vi "Agilent DSO1000 Series Acquire Multiple Waveforms.vi"() -> ()   [LabVIEW 2010]
doc: "This example shows how to configure multiple channels and acquire waveforms from multiple channels."
uses:
  <instrlib>/Agilent DSO1000 Series/Public/Data/Read Waveform (Multiple).vi
  <instrlib>/Agilent DSO1000 Series/Agilent DSO1000 Series.lvlib
panel:
  in  "Probe Attenuation (3: 1X)":u16(ring)=3 items=["0.001X", "0.01X", "0.1X", "1X", "10X", "100X", "1000X"]
  in  "Probe Attenuation (3: 1X)":u16(ring)=3 items=["0.001X", "0.01X", "0.1X", "1X", "10X", "100X", "1000X"]
  in  "Channel (1: Channel 1)":u16(ring)=2 items=["Channel 1"=1, "Channel 2"=2, "Channel 3"=3, "Channel 4"=4]
  in  "Channel (1: Channel 1)":u16(ring)=1 items=["Channel 1"=1, "Channel 2"=2, "Channel 3"=3, "Channel 4"=4]
  in  "Maximum Time (10000 ms)":u32=10000
  in  "Vertical Coupling (1: DC)":u16(ring)=1 items=["AC", "DC", "Ground"]
  in  "Vertical Coupling (1: DC)":u16(ring)=1 items=["AC", "DC", "Ground"]
  out "Waveform Data":waveform(dbl)[](graph)
  in  "VISA resource name":refnum<visa-resource-name>
  # "(c) 2009 National Instruments.  ALL RIGHTS RESERVED."
  # "Channel A"
  # "Channel B"
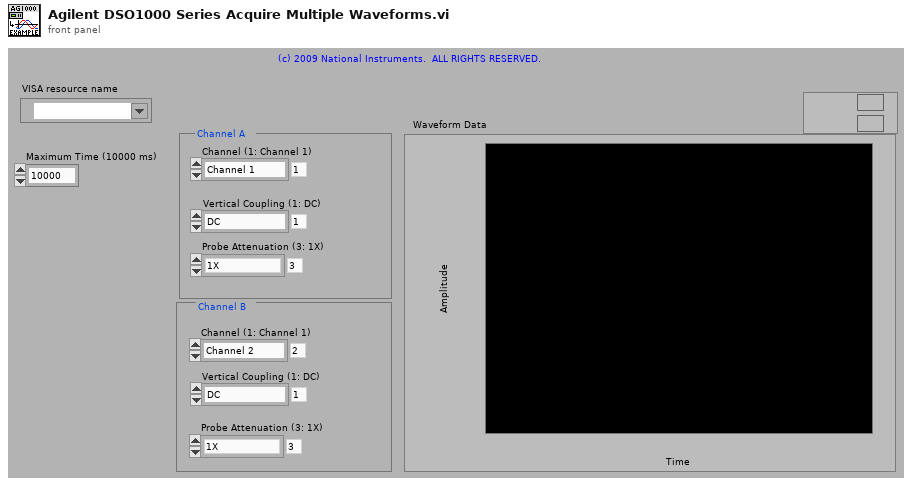
[diagram p1: front panel]
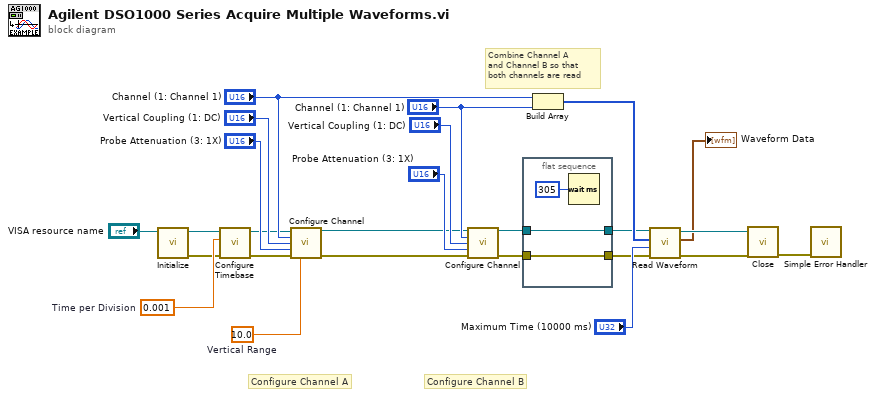
[diagram p0: block diagram]
diagram:
  w21 = 0.001  # Time per Division
  w9 = 10.0  # Vertical Range
  # "Combine Channel A\nand Channel B so that\nboth channels are read"
  # "Configure Channel B"
  # "Configure Channel A"
  n1 = call <instrlib>:"Initialize.vi"("VISA resource name"="VISA resource name") -> ("error out"=w7:errorcluster, "VISA resource name out"=w8:refnum<visa-resource-name>)  [unwired: 9 in]
  n2 = call <instrlib>:"Configure Timebase.vi"("error in (no error)"=w7, "Timebase (1E-6 s)"=w21, "VISA resource name"=w8) -> ("error out"=w5:errorcluster, "VISA resource name out"=w6:refnum<visa-resource-name>)  [unwired: 7 in]
  n3 = call <instrlib>:"Configure Channel.vi"("VISA resource name"=w6, "Channel (1: Channel 1)"="Channel (1: Channel 1)", "Vertical Coupling (1: DC)"="Vertical Coupling (1: DC)", "Probe Attenuation (3: 1X)"="Probe Attenuation (3: 1X)", "error in (no error)"=w5, "Vertical Range (10.0 V)"=w9) -> ("VISA resource name out"=w11:refnum<visa-resource-name>, "error out"=w10:errorcluster)  [unwired: 8 in]
  n4 = call <instrlib>:"Configure Channel.vi"("VISA resource name"=w11, "Channel (1: Channel 1)"="Channel (1: Channel 1)", "Vertical Coupling (1: DC)"="Vertical Coupling (1: DC)", "Probe Attenuation (3: 1X)"="Probe Attenuation (3: 1X)", "error in (no error)"=w10) -> ("VISA resource name out"=w4:refnum<visa-resource-name>, "error out"=w2:errorcluster)  [unwired: 9 in]
  n5 = flat-sequence {
    tunnel: w4 -> [w28]
    tunnel: [w28] -> w3
    tunnel: w2 -> [w27]
    tunnel: [w27] -> w1
    frame #0 {
      n6 = Wait (ms)(milliseconds to wait=u32 305) -> ()  [unwired: 1 out]
    }
  }
  n7 = Build Array("Channel (1: Channel 1)", "Channel (1: Channel 1)") -> (w16:u16[])
  n8 = call-poly <instrlib>:"Read Waveform.vi"("error in (no error)"=w1, "Maximum Time (10000 ms)"="Maximum Time (10000 ms)", "Channels"=w16, "VISA resource name"=w3) -> ("error out"=w18:errorcluster, "Waveform Data"=→"Waveform Data":waveform(dbl)[], "VISA resource name out"=w20:refnum<visa-resource-name>)  [unwired: 5 in]
  n9 = call <instrlib>:"Close.vi"("error in (no error)"=w18, "VISA resource name"=w20) -> ("error out"=w24:errorcluster)  [unwired: 9 in]
  n10 = call <vilib>:"Simple Error Handler.vi"("error in (no error)"=w24) -> ()  [unwired: 4 in, 5 out]
